vi "Delete Dynamic RPTID File.vi"(8 "error in (no error)":errorcluster) -> (0 "error out":errorcluster)   [LabVIEW 2020, in "SECS Communication.lvlib" / "SECS Data Class.lvclass"]
uses:
  SECS Data Class.lvclass
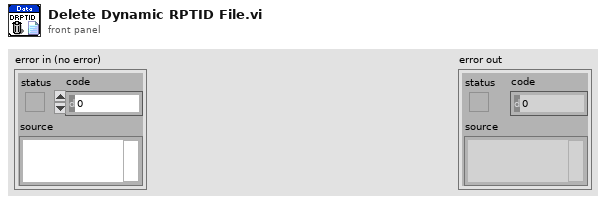
[diagram p1: front panel]
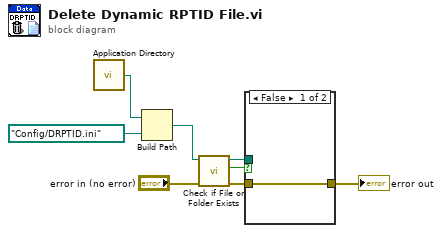
[diagram p0: block diagram]
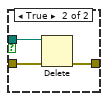
[diagram p2: hidden frame]
diagram:
  n1 = call <vilib>:"Application Directory.vi"() -> ("Application Directory"=w8:path)
  n2 = Build Path(base path=w8, name or relative path=path "Config/DRPTID.ini") -> (appended path=w4:path)
  n3 = call <vilib>:"Check if File or Folder Exists.vi"("error in (no error)"="error in (no error)", "path"=w4) -> ("error out"=w3:errorcluster, "file or folder exists?"=w1:bool, "dup path"=w2:path)  [unwired: 7 in]
  n4 = case shown="False" w1 {
    tunnel: [w9 w12] -> w6
    tunnel: w3 -> [w9 w11]
    tunnel: w2 -> [_ w10]
    frame False {
    }
    frame True {
      n5 = Delete(path (use dialog)=w10, error in=w11) -> (error out=w12:errorcluster)  [unwired: 3 in, 2 out]
    }
  }
  "error out" <- w6
